vi "捆绑力曲线C.vi"(1 "力数组":sgl[](array[numeric]), 3 "Pr":T1={"选择"=enum."Fx", "系数x"=1.0, "系数+"=1.0, "上限"=4.3, "下限"=3.7, "Ymax"=50.0, "Ymin"=-50.0, "点数"=1000.0, "锁系数x"=1.0, "锁上限"=0.4, "锁下限"=0.6, "锁系数+"=1.0, "起点"=0.20000000298023224, "终点"=0.6499999761581421, "锁起点"=0.05000000074505806, "锁终点"=0.20000000298023224, "上参考"=4.3, "下参考"=3.7, "基准"=3.7} {"系数+" format="%.3f"; "基准" format="%.2f"; "下参考" format="%.2f"; "上参考" format="%.2f"; "锁终点" format="%.2f"; "锁起点" format="%.2f"; "终点" format="%.2f"; "起点" format="%.2f"; "锁系数+" format="%.3f"; "锁下限" format="%.2f"; "锁上限" format="%.2f"; "锁系数x" format="%.3f"; "下限" format="%.2f"; "上限" format="%.2f"; "系数x" format="%.3f"}) -> (0 "历史数据":T2(array[cluster]))   [LabVIEW 2018]
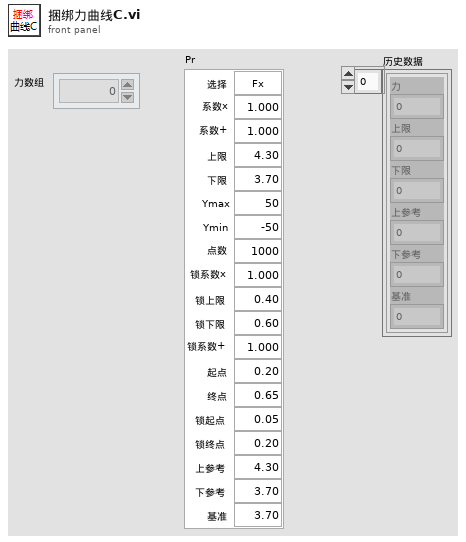
[diagram p1: front panel]
types:
  T1 = cluster{"选择":enum16{"Fx", "Fy", "Fz", "Mx", "My", "Mz"}, "系数x":sgl, "系数+":sgl, "上限":sgl, "下限":sgl, "Ymax":dbl, "Ymin":dbl, "点数":dbl, "锁系数x":sgl, "锁上限":sgl, "锁下限":sgl, "锁系数+":sgl, "起点":dbl, "终点":dbl, "锁起点":dbl, "锁终点":dbl, "上参考":sgl, "下参考":sgl, "基准":sgl}
  T2 = cluster{"力":sgl, "上限":sgl, "下限":sgl, "上参考":sgl, "下参考":sgl, "基准":sgl}[]
  T3 = cluster{"力":sgl, "上限":sgl, "下限":sgl, "上参考":sgl, "下参考":sgl, "基准":sgl}
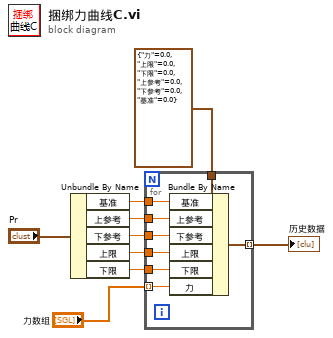
[diagram p0: block diagram]
diagram:
  n1 = Unbundle By Name("Pr") -> ("基准"=w6:sgl, "上参考"=w5:sgl, "下参考"=w4:sgl, "上限"=w3:sgl, "下限"=w2:sgl)
  n2 = for {
    tunnel: "力数组" -> [w17] mode=indexing
    tunnel: [w16] -> w8 mode=indexing
    tunnel: T3 {"力"=0.0, "上限"=0.0, "下限"=0.0, "上参考"=0.0, "下参考"=0.0, "基准"=0.0} -> [w15]
    tunnel: w6 -> [w14]
    tunnel: w5 -> [w13]
    tunnel: w4 -> [w12]
    tunnel: w3 -> [w11]
    tunnel: w2 -> [w10]
    n3 = Bundle By Name(cluster=w15, "基准"=w14, "上参考"=w13, "下参考"=w12, "上限"=w11, "下限"=w10, "力"=w17) -> (w16:T3)
  }
  "历史数据" <- w8
